vi "GetParam.vi"(8 "error in (no error)":errorcluster caption="entrée d'erreur (pas d'erreur)", 11 "lfw_pairs.lvclass":refnum<class "lfw_pairs.lvclass">) -> (0 "error out":errorcluster caption="sortie d'erreur", 2 "fetch_lfw_pairs":T1={"subset"="train", "funneled"=TRUE, "resize"=0.5, "color"=FALSE, "slice_"={"Cluster"={"height"=70, "width"=195}, "Cluster 2"={"height"=78, "width"=172}}, "download_if_missing"=TRUE, "Returns"="Data"}, 3 "lfw_pairs.lvclass":refnum<class "lfw_pairs.lvclass">)   [LabVIEW 2020, in "lfw_pairs.lvclass"]
doc: "Get parameters"
uses:
  lfw_pairs.lvclass
  lfw_pairs.lvclass/lfw_pairs.ctl
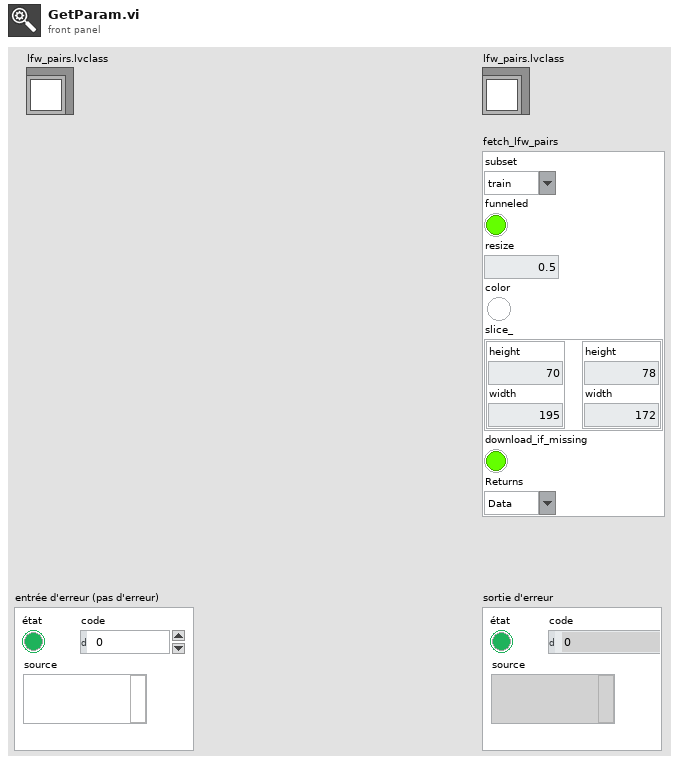
[diagram p1: front panel]
types:
  T1 = cluster{"subset":string, "funneled":bool, "resize":dbl, "color":bool, "slice_":cluster{"Cluster":cluster{"height":u32, "width":u32}, "Cluster 2":cluster{"height":u32, "width":u32}}, "download_if_missing":bool, "Returns":string}
  T2 = cluster{"subset":string, "funneled":bool, "resize":dbl, "color":bool, "slice_":cluster{"Cluster":cluster{"height":u32, "width":u32}, "Cluster 2":cluster{"height":u32, "width":u32}}, " download_if_missing ":bool, "Returns":string}
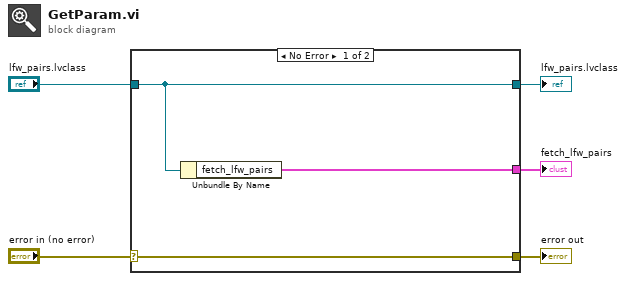
[diagram p0: block diagram]
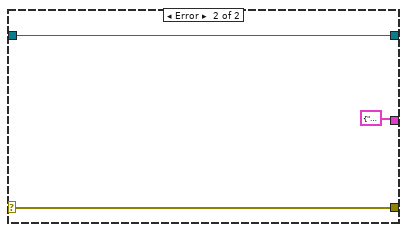
[diagram p2: hidden frame]
diagram:
  n1 = case shown="No Error" "error in (no error)" {
    selector: "error in (no error)" -> [w8 w10]
    tunnel: [w8 w10] -> w4
    tunnel: [w7 w11] -> w2
    tunnel: "lfw_pairs.lvclass" -> [w7 w11]
    tunnel: [w6 T2 {"subset"="", "funneled"=FALSE, "resize"=0.0, "color"=FALSE, "slice_"={"Cluster"={"height"=0, "width"=0}, "Cluster 2"={"height"=0, "width"=0}}, " download_if_missing "=FALSE, "Returns"=""} ("fetch_lfw_pairs")] -> w1
    frame No Error {
      n2 = Unbundle By Name(w7) -> ("fetch_lfw_pairs"=w6:T2)
    }
    frame Error {
    }
  }
  "error out" <- w4
  "lfw_pairs.lvclass" <- w2
  "fetch_lfw_pairs" <- w1
